vi "maintenanceBLE.vi"(11 "Shared_strings":string[][](array[string])) -> ()   [LabVIEW 2018]
uses:
  Global Variables.vi
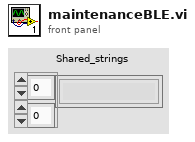
[diagram p1: front panel]
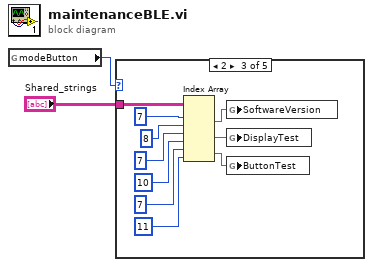
[diagram p0: block diagram]
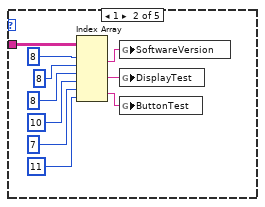
[diagram p3: hidden frame]
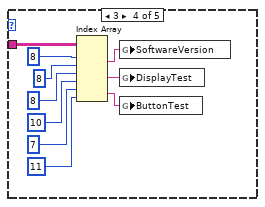
[diagram p4: hidden frame]
diagram:
  n1 = global read "Global Variables.vi" "modeButton"() -> (w1:i32)
  n2 = case shown="2" w1 {
    tunnel: "Shared_strings" -> [_ w12 w19 w23 _]
    frame 0, Default {
    }
    frame 1 {
      n3 = Index Array(array=w12, index (row) #1=8 ("index (row)"), index (col) #1=8 ("disabled index (col)"), index (row) #2=8 ("index (row)"), index (col) #2=10 ("disabled index (col)"), index (row) #3=7 ("index (row)"), index (col) #3=11 ("disabled index (col)")) -> (element #1=w11:string, element #2=w8:string, element #3=w7:string)
      n4 = global write "Global Variables.vi" "SoftwareVersion"(w11) -> ()
      n5 = global write "Global Variables.vi" "DisplayTest"(w8) -> ()
      n6 = global write "Global Variables.vi" "ButtonTest"(w7) -> ()
    }
    frame 2 {
      n7 = Index Array(array=w19, index (row) #1=7 ("index (row)"), index (col) #1=8 ("disabled index (col)"), index (row) #2=7 ("index (row)"), index (col) #2=10 ("disabled index (col)"), index (row) #3=7 ("index (row)"), index (col) #3=11 ("disabled index (col)")) -> (element #1=w22:string, element #2=w18:string, element #3=w17:string)
      n8 = global write "Global Variables.vi" "SoftwareVersion"(w22) -> ()
      n9 = global write "Global Variables.vi" "DisplayTest"(w18) -> ()
      n10 = global write "Global Variables.vi" "ButtonTest"(w17) -> ()
    }
    frame 3 {
      n11 = Index Array(array=w23, index (row) #1=8 ("index (row)"), index (col) #1=8 ("disabled index (col)"), index (row) #2=8 ("index (row)"), index (col) #2=10 ("disabled index (col)"), index (row) #3=7 ("index (row)"), index (col) #3=11 ("disabled index (col)")) -> (element #1=w32:string, element #2=w29:string, element #3=w28:string)
      n12 = global write "Global Variables.vi" "SoftwareVersion"(w32) -> ()
      n13 = global write "Global Variables.vi" "DisplayTest"(w29) -> ()
      n14 = global write "Global Variables.vi" "ButtonTest"(w28) -> ()
    }
    frame 4 {
      # "PowerGlyph"
    }
  }
